vi "GatheringSerialPortNames.vi"(9 "old Name":string) -> (1 "name":string)   [LabVIEW 2016]
panel:
  in  "done":bool
  in  "Name":string
  in  "Refresh":bool
  in  "Name It":bool
  in  "Ports":i32(listbox)
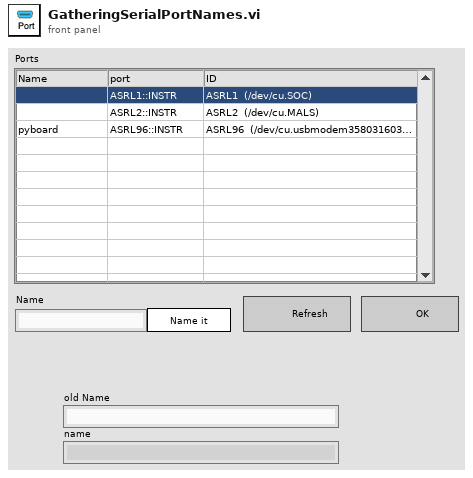
[diagram p1: front panel]
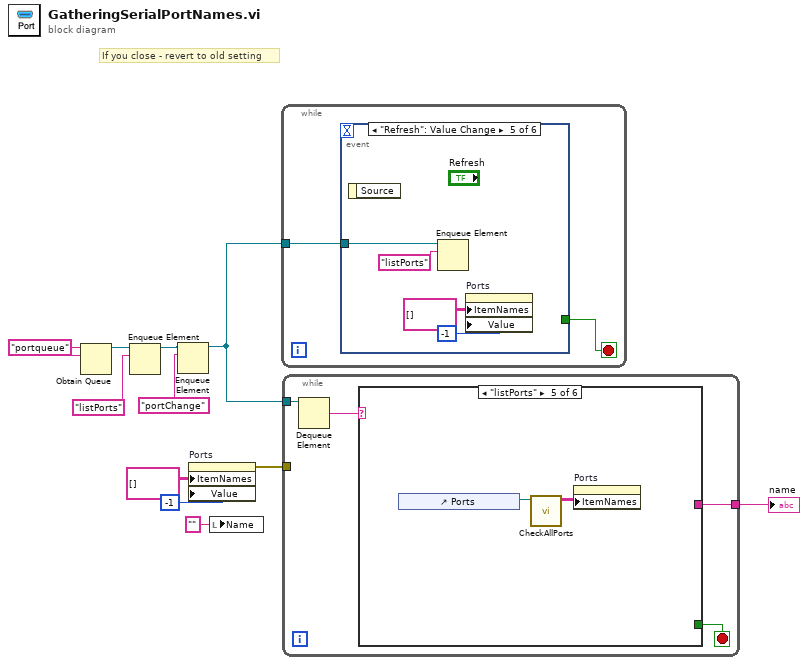
[diagram p0: block diagram]
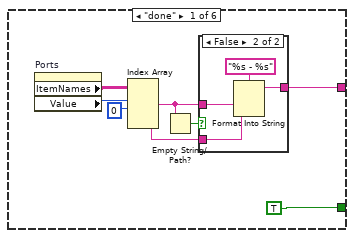
[diagram p2: hidden frame]
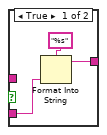
[diagram p3: hidden frame]
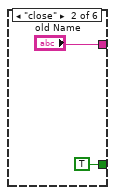
[diagram p4: hidden frame]
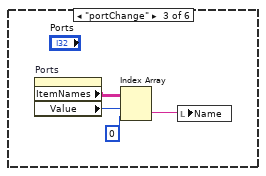
[diagram p5: hidden frame]
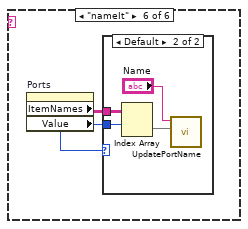
[diagram p7: hidden frame]
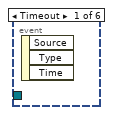
[diagram p9: hidden frame]
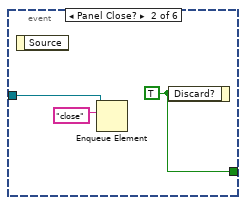
[diagram p10: hidden frame]
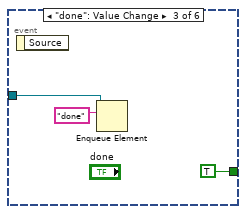
[diagram p11: hidden frame]
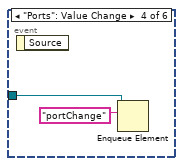
[diagram p12: hidden frame]
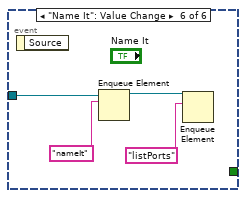
[diagram p13: hidden frame]
diagram:
  w9 = "portqueue" ("name (unnamed)")
  # "If you close - revert to old setting"
  n1 = Obtain Queue(name (unnamed)=w9, element data type=w9) -> (queue out=w11:refnum<queue>)  [unwired: 3 in, 2 out]
  n2 = Enqueue Element(queue=w11, element="listPorts") -> (queue out=w7:refnum<queue>)  [unwired: 2 in, 2 out]
  n3 = Enqueue Element(queue=w7, element="portChange") -> (queue out=w6:refnum<queue>)  [unwired: 2 in, 2 out]
  n4 = property on="Ports" class="MCListbox (strict)"("ItemNames"=string[][] [] ("Item Names"), "Value"=-1 ("Ports")) -> (error out=w1:errorcluster)  [unwired: 2 in, 1 out]
  n5 = local write "Name"("" ("Name")) -> ()
  n6 = while {
    tunnel: w6 -> [w12]
    stop <- w13 stop-if-true
    n7 = event shown="[4] \"Refresh\": Value Change" {
      selector: _ -> [_ _ _ _ _ _]
      dyn-events: _ -> [_ _ _ _ _ _]
      timeout: _ -> [_ _ _ _ _ _]
      tunnel: [_ w16 TRUE ("Discard?") _ _ _] -> w13
      tunnel: w12 -> [_ w14 w18 w20 w24 w27]
      event Timeout {
        n8 = event-data() -> ()  [unwired: 1 in, 3 out]
      }
      event Panel Close? {
        w16 = TRUE ("Discard?")
        n9 = event-data() -> ()  [unwired: 1 in, 1 out]
        n10 = Enqueue Element(queue=w14, element="close") -> ()  [unwired: 2 in, 3 out]
        n11 = event-data("Discard?"=w16) -> ()  [unwired: 1 in, 1 out]
      }
      event "done": Value Change {
        n12 = event-data() -> ()  [unwired: 1 in, 1 out]
        n13 = Enqueue Element(queue=w18, element="done") -> ()  [unwired: 2 in, 3 out]
      }
      event "Ports": Value Change {
        n14 = event-data() -> ()  [unwired: 1 in, 1 out]
        n15 = Enqueue Element(queue=w20, element="portChange") -> ()  [unwired: 2 in, 3 out]
      }
      event "Refresh": Value Change {
        n16 = event-data() -> ()  [unwired: 1 in, 1 out]
        n17 = Enqueue Element(queue=w24, element="listPorts") -> ()  [unwired: 2 in, 3 out]
        n18 = property on="Ports" class="MCListbox (strict)"("ItemNames"=string[][] [] ("Item Names"), "Value"=-1 ("Ports")) -> ()  [unwired: 2 in, 2 out]
      }
      event "Name It": Value Change {
        n19 = event-data() -> ()  [unwired: 1 in, 1 out]
        n20 = Enqueue Element(queue=w27, element="nameIt") -> (queue out=w26:refnum<queue>)  [unwired: 2 in, 2 out]
        n21 = Enqueue Element(queue=w26, element="listPorts") -> ()  [unwired: 2 in, 3 out]
      }
    }
  }
  n22 = while {
    tunnel: w6 -> [w33]
    tunnel: [w30] -> w2
    tunnel: w1 -> [_]
    stop <- w31 stop-if-true
    n23 = Dequeue Element(queue=w33) -> (element=w32:string)  [unwired: 2 in, 3 out]
    n24 = case shown="\"listPorts\"" w32 {
      tunnel: [TRUE TRUE _ _ _ _] -> w31
      tunnel: [w34 "old Name" _ _ _ _] -> w30
      frame "done" {
        n25 = property on="Ports" class="MCListbox (strict)"() -> ("ItemNames"=w40:string[][], "Value"=w39:i32)  [unwired: 2 in, 2 out]
        n26 = Index Array(array=w40, index (row) #1=w39, index (col) #1=0 ("disabled index (col)")) -> (element #1=w36:string, element #2=w35:string)  [unwired: 2 in]
        n27 = Empty String/Path?(string/path=w36) -> (empty?=w38:bool)
        n28 = case shown="False" w38 {
          tunnel: w35 -> [w42 w47]
          tunnel: [w43 w46] -> w34
          tunnel: w36 -> [_ w45]
          frame True {
            n29 = Format Into String(format string="%s", w42) -> (resulting string=w43:string)  [unwired: 2 in, 1 out]
          }
          frame False {
            n30 = Format Into String(format string="%s - %s", w45, w47) -> (resulting string=w46:string)  [unwired: 2 in, 1 out]
          }
        }
      }
      frame "close" {
      }
      frame "portChange" {
        n31 = property on="Ports" class="MCListbox (strict)"() -> ("ItemNames"=w54:string[][], "Value"=w52:i32)  [unwired: 2 in, 2 out]
        n32 = Index Array(array=w54, index (row)=w52, index (col)=0 ("disabled index (col)")) -> (element=w51:string)
        n33 = local write "Name"(w51) -> ()
      }
      frame Default {
      }
      frame "listPorts" {
        n34 = control-ref of="Ports"() -> (w55:refnum<vi>)
        n35 = call "CheckAllPorts.vi"("Ports"=w55) -> ("Ports"=w56:string[][])  [unwired: 10 in]
        n36 = property on="Ports" class="MCListbox (strict)"("ItemNames"=w56) -> ()  [unwired: 2 in, 2 out]
      }
      frame "nameIt" {
        n37 = property on="Ports" class="MCListbox (strict)"() -> ("ItemNames"=w58:string[][], "Value"=w57:i32)  [unwired: 2 in, 2 out]
        n38 = case shown="Default" w57 {
          tunnel: w58 -> [_ w62]
          tunnel: w57 -> [_ w61]
          frame -1 {
          }
          frame Default {
            n39 = Index Array(array=w62, index (row)=w61) -> (element=w60:string[])  [unwired: 1 in]
            n40 = call "UpdatePortName.vi"("ItemNames"=w60, "Name"="Name") -> ()  [unwired: 10 in]
          }
        }
      }
    }
  }
  "name" <- w2
